vi "Get Size.vi"(0 "image in":refnum<class "MSC Image.lvclass">, 5 "error in (no error)":errorcluster) -> (14 "image out":refnum<class "MSC Image.lvclass">, 15 "Size":T1, 19 "error out":errorcluster)   [LabVIEW 2014, in "MSC Image.lvclass"]
doc: "Returns the image size."
uses:
  MSC Image.lvclass
  controls/Size.ctl
  MSC Image.lvclass/MSC Image.ctl
panel:
  out "Rows":i32
  out "Cols":i32
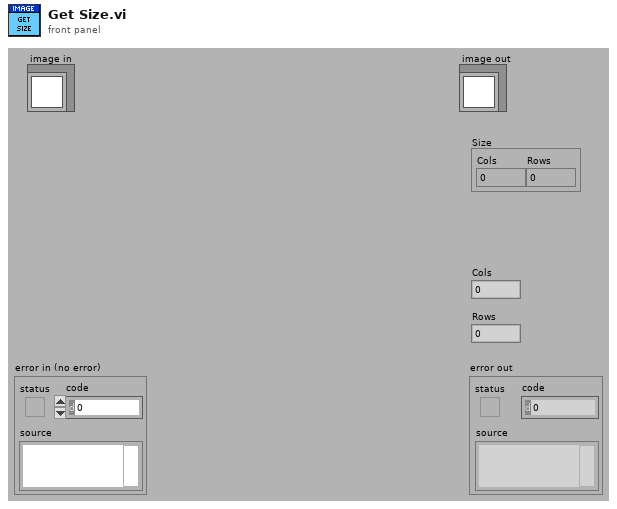
[diagram p1: front panel]
types:
  T1 = typedef "MSC Image.lvclass/Size.ctl" = cluster{"Cols":i32, "Rows":i32}
  T2 = typedef "Image.ctl" = cluster{"Pointer":u64, "Size":T3, "Image Type":T4, "Time Stamp":timestamp, "Variant":variant}
  T3 = typedef "Size.ctl" = cluster{"Cols":i32, "Rows":i32}
  T4 = typedef "Image Type.ctl" = i32
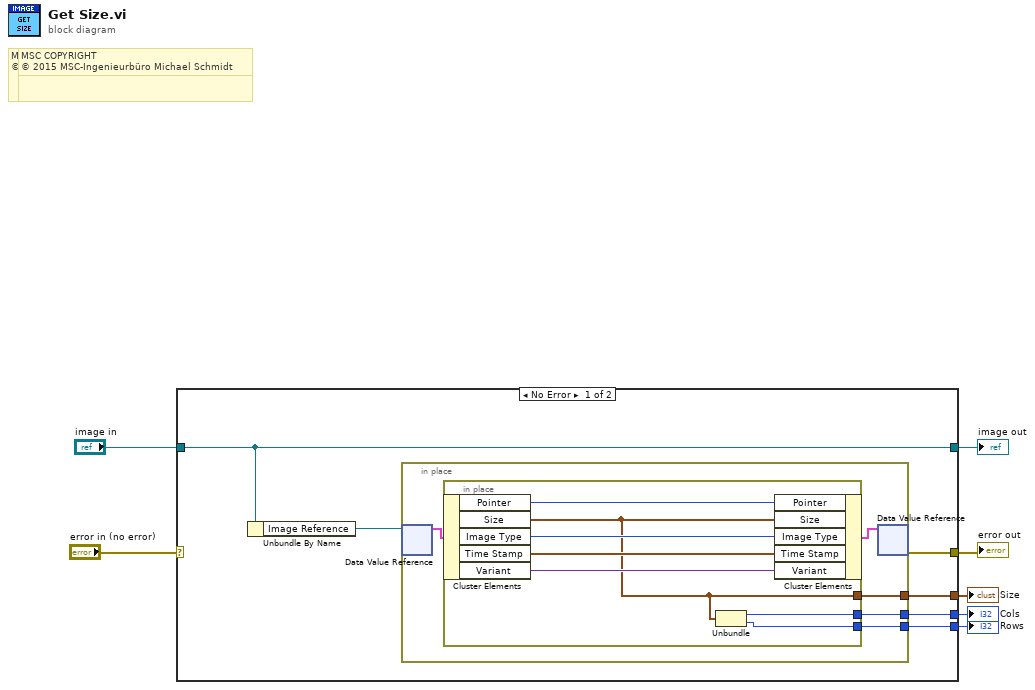
[diagram p0: block diagram]
diagram:
  # "MSC COPYRIGHT\n© 2016 MSC-Ingenieurbüro Michael Schmidt"
  # "MSC COPYRIGHT\n© 2016 MSC-Ingenieurbüro Michael Schmidt"
  # "MSC COPYRIGHT\n© 2015 MSC-Ingenieurbüro Michael Schmidt"
  # "MSC COPYRIGHT\n© 2015 MSC-Ingenieurbüro Michael Schmidt"
  n1 = case shown="No Error" "error in (no error)" {
    selector: "error in (no error)" -> [_ w27]
    tunnel: [w11 w27] -> w6
    tunnel: [w13 w26] -> w4
    tunnel: "image in" -> [w13 w26]
    tunnel: [w10 _] -> w3
    tunnel: [w9 _] -> w2
    tunnel: [w8 _] -> w1
    frame No Error {
      n2 = Unbundle By Name(w13) -> ("Image Reference"=w12:refnum<data-value>)
      n3 = in-place {
        in-place-border: [w16] -> w10
        in-place-border: [w15] -> w9
        in-place-border: [w14] -> w8
        n4 = in-place-dvr #1(w12) -> (w17:T2)  [unwired: 1 out]
        n5 = in-place {
          in-place-border: [w21] -> w16
          in-place-border: [w20] -> w15
          in-place-border: [w19] -> w14
          n6 = in-place-cluster #2(w17) -> ("Pointer"=w25:u64, "Size"=w21:T3, "Image Type"=w24:T4, "Time Stamp"=w22:timestamp, "Variant"=w23:variant)
          n7 = Unbundle(w21) -> ("Cols"=w20:i32, "Rows"=w19:i32)
          n8 = in-place-cluster #2("Pointer"=w25, "Size"=w21, "Image Type"=w24, "Time Stamp"=w22, "Variant"=w23) -> (w18:T2)
        }
        n9 = in-place-dvr #1(w18) -> (w11:errorcluster)  [unwired: 1 out]
      }
    }
    frame Error {
    }
  }
  "error out" <- w6
  "image out" <- w4
  "Size" <- w3
  "Cols" <- w2
  "Rows" <- w1
